vi "Call Matlab Function.vi"(8 "error in (no error)":errorcluster, 9 "Matlab Param Array":cluster{"Name":string, "Data":variant}[](array[cluster]), 10 "Function name":string, 11 "TCP Network Connection Refnum":refnum<k5>) -> (0 "error out":errorcluster, 1 "Return value struct":cluster{"Name":string, "Data":variant}[](array[cluster]), 2 "Return value I32":i32, 3 "connection ID out":refnum<k5>)   [LabVIEW 2014, in "Matlab API.lvlib"]
uses:
  Matlab API.lvlib
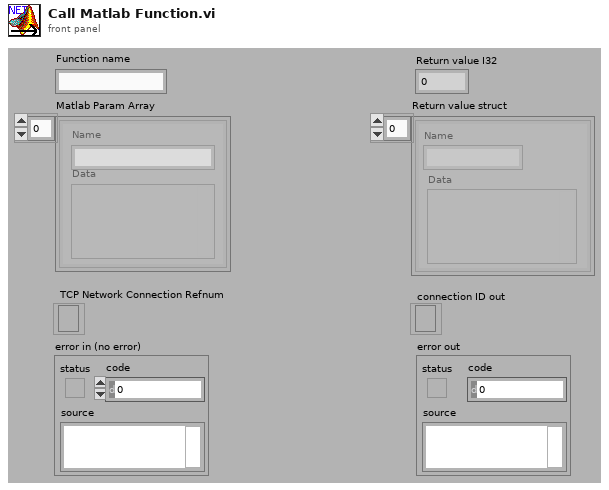
[diagram p1: front panel]
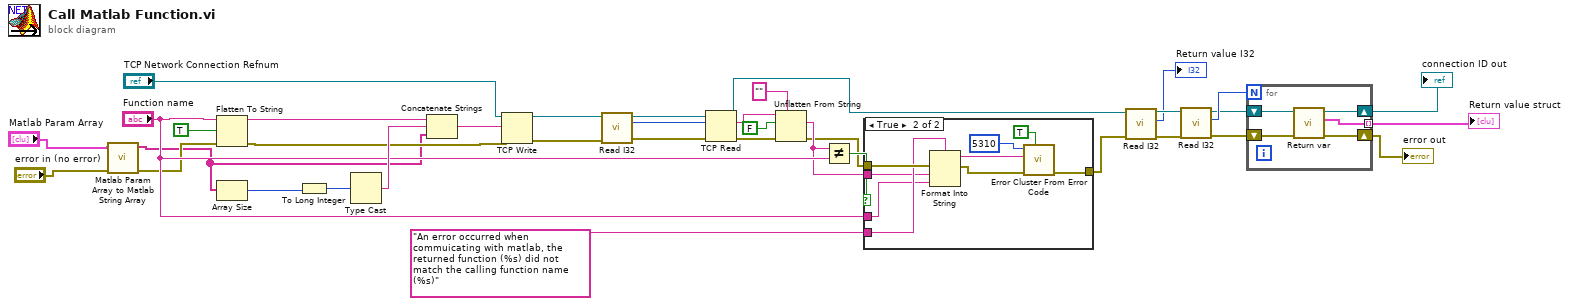
[diagram p0: block diagram]
diagram:
  n1 = call "Matlab Param Array to Matlab String Array.vi"("error in"="error in (no error)", "Matlab Param Array"="Matlab Param Array") -> ("error out"=w8:errorcluster, "Matlab Strings"=w7:string[])  [unwired: 8 out]
  n2 = Flatten To String(anything="Function name", prepend array or string size? (T)=TRUE, error in (no error)=w8) -> (data string=w36:string, error out=w31:errorcluster)  [unwired: 2 out]
  n3 = Array Size(array=w7) -> (size(s)=w34:i32)
  n4 = To Long Integer(number=w34) -> (32bit integer=w33:i32)
  n5 = Type Cast(x=w33) -> (*(type *) &x=w35:string)  [unwired: 1 out]
  n6 = Concatenate Strings(w36, w35, w7) -> (w24:string)
  n7 = TCP Write(connection ID="TCP Network Connection Refnum", data in=w24, error in (no error)=w31) -> (connection ID out=w22:refnum<k5>, error out=w6:errorcluster)  [unwired: 2 out]
  n8 = call "Read I32.vi"("error in (no error)"=w6, "connection ID"=w22) -> ("error out"=w3:errorcluster, "value"=w21:i32, "connection ID out"=w20:refnum<k5>)  [unwired: 7 out]
  n9 = TCP Read(connection ID=w20, bytes to read=w21, error in (no error)=w3) -> (connection ID out=w18:refnum<k5>, data out=w19:string, error out=w4:errorcluster)  [unwired: 2 out]
  n10 = Unflatten From String(type="", binary string=w19, data includes array or string size? (T)=FALSE, error in (no error)=w4) -> (value=w25:string, error out=w10:errorcluster)  [unwired: 2 out]
  n11 = Not Equal?(x=w25, y="Function name") -> (x != y?=w28:bool)
  n12 = case shown="True" w28 {
    tunnel: w10 -> [w38 w46]
    tunnel: "Function name" -> [_ w44]
    tunnel: "An error occurred when commuicating with matlab, the returned function (%s) did not match the calling function name (%s)" ("initial string") -> [_ w45]
    tunnel: w25 -> [_ w43]
    tunnel: [w38 w39] -> w5
    frame False {
    }
    frame True {
      n13 = Format Into String(format string=w45, error in=w46, w43, w44) -> (resulting string=w42:string, error out=w41:errorcluster)  [unwired: 1 in]
      n14 = call <vilib>:"Error Cluster From Error Code.vi"("show call chain? (False)"=TRUE, "error in (no error)"=w41, "error message (\"\")"=w42, "error code (0)"=5310) -> ("error out"=w39:errorcluster)  [unwired: 5 out]
    }
  }
  n15 = call "Read I32.vi"("error in (no error)"=w5, "connection ID"=w18) -> ("error out"=w17:errorcluster, "value"=→"Return value I32":i32, "connection ID out"=w15:refnum<k5>)  [unwired: 7 out]
  n16 = call "Read I32.vi"("error in (no error)"=w17, "connection ID"=w15) -> ("error out"=w16:errorcluster, "value"=w13:i32, "connection ID out"=w12:refnum<k5>)  [unwired: 7 out]
  n17 = for {
    N: w13 -> [_]
    shift-right: [w48] -> w1
    shift-left: w16 -> [w51]
    tunnel: [w50] -> w23 mode=indexing
    shift-right: [w49] -> w11
    shift-left: w12 -> [w52]
    n18 = call "Return var.vi"("error in (no error)"=w51, "connection ID"=w52) -> ("error out"=w48:errorcluster, "output cluster"=w50:cluster{"Name":string, "Data":variant}, "connection ID out"=w49:refnum<k5>)  [unwired: 7 out]
  }
  "connection ID out" <- w11
  "error out" <- w1
  "Return value struct" <- w23
